vi "Drive Threshold and Half.vi"(0 "X In":dbl, 1 "Drive refnum name":string="RobotDrive", 2 "Send to DB Name":string="Numeric Array", 5 "Y In":dbl, 7 "R In":dbl, 9 "Speed Toggle":bool, 11 "Error In":errorcluster) -> (15 "Error Out":errorcluster)   [LabVIEW 2014]
uses:
  <vilib>/Rock Robotics/WPI/RobotDrive/WPI_RobotDriveGetSetRefNum.vi
  <vilib>/Rock Robotics/WPI/RobotDrive/WPI_RobotDriveMecanumDrive_Cartesian.vi
  <vilib>/Rock Robotics/Network Tables/SD Write Numeric Array.vi
panel:
  out "X Original":dbl
  out "X Threshold":dbl
  out "Y Original":dbl
  out "Y Threshold":dbl
  out "R Original":dbl
  out "R Threshold":dbl
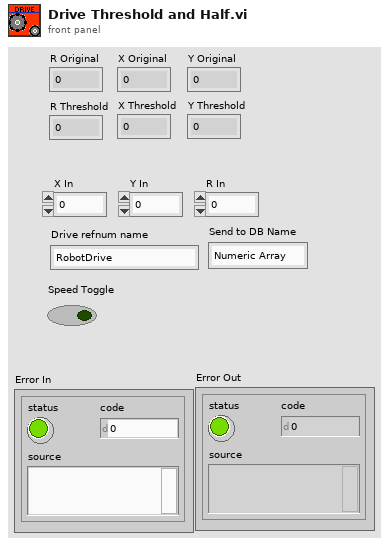
[diagram p1: front panel]
types:
  T1 = typedef "WPI_RobotDriveDevRef.ctl" = cluster{"DevStatus":errorcluster, "Motors[]":T2[], "Square Inputs":bool, "Max Output":dbl}
  T2 = typedef "WPI_MotorControlDeviceRef.ctl" = cluster{"DeviceStatus":errorcluster, "Type":T3, "PWM":cluster{"Controller":T4, "PWM Channel":T5, "DeadBand":T6}, "CAN":cluster{"Device Number":u8, "Control Mode":T7, "Semaphore":T8, "Max Vout":dbl, "TalonSRX Control Mode":T9}, "Invert":bool, "TransformRef":T10, "InvTransformRef":T10}
  T3 = typedef "WPI_MotorControlType.ctl" = enum16{"PWM", "CAN", "CANTalonSRX"}
  T4 = typedef "FPGA_TypedefDigitalModule.ctl" = enum16{"Controller 1"}
  T5 = typedef "FPGA_DIOPWMChannel.ctl" = enum8{"PWM 0", "PWM 1", "PWM 2", "PWM 3", "PWM 4", "PWM 5", "PWM 6", "PWM 7", "PWM 8", "PWM 9", "PWM MXP 0", "PWM MXP 1", "PWM MXP 2", "PWM MXP 3", "PWM MXP 4", "PWM MXP 5", "PWM MXP 6", "PWM MXP 7", "PWM MXP 8", "PWM MXP 9", "Invalid"}
  T6 = typedef "WPI_PWMDeadband.ctl" = cluster{"Name":string, "maxPositivePwm":i32, "minPositivePwm":i32, "centerPwm":i32, "maxNegativePwm":i32, "minNegativePwm":i32, "angularRange":u16}
  T7 = typedef "WPI_CANJaguar_ControlMode.ctl" = enum8{"Percent VBus", "Current", "Speed", "Position", "Voltage"}
  T8 = typedef "Semaphore RefNum" = refnum<k1>
  T9 = typedef "WPI_CANTalonSRX_APIControlMode.ctl" = enum8{"Percent VBus", "Speed", "Position", "Slave", "Unchanged / Invalid"}
  T10 = typedef "WPI_PWMTransform_ConPane.ctl" = refnum<vi>
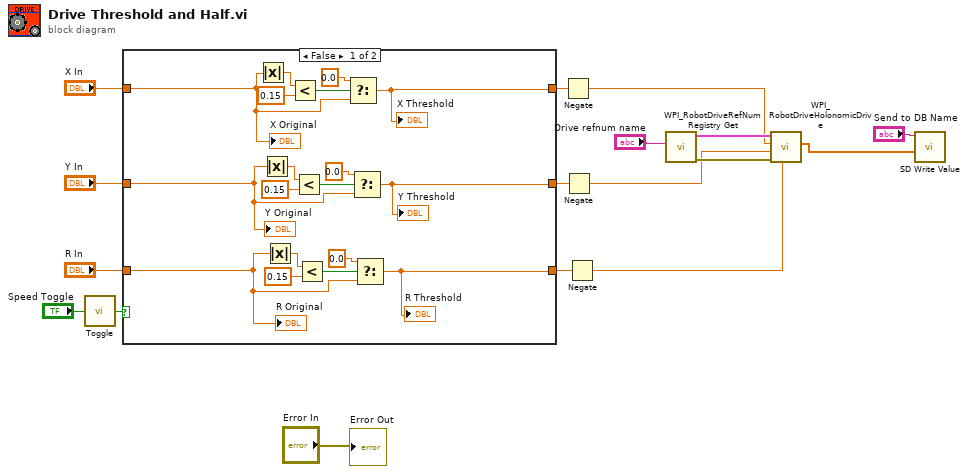
[diagram p0: block diagram]
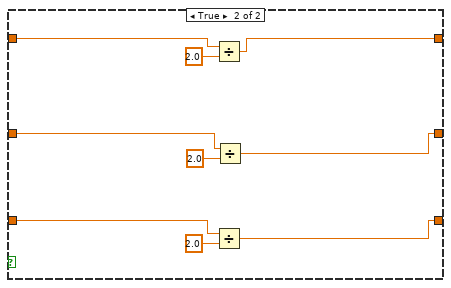
[diagram p2: hidden frame]
diagram:
  n1 = call "Toggle.vi"("Input"="Speed Toggle") -> ("Output"=w17:bool)
  n2 = case shown="False" w17 {
    tunnel: [w30 w38] -> w16
    tunnel: "X In" -> [w31 w39]
    tunnel: "Y In" -> [w25 w40]
    tunnel: [w24 w37] -> w11
    tunnel: "R In" -> [w19 w41]
    tunnel: [w18 w36] -> w10
    frame False {
      n3 = Absolute Value(x=w31) -> (abs(x)=w35:dbl)
      n4 = Absolute Value(x=w25) -> (abs(x)=w29:dbl)
      n5 = Absolute Value(x=w19) -> (abs(x)=w20:dbl)
      n6 = Less?(x=w35, y=0.15) -> (x < y?=w33:bool)
      n7 = Less?(x=w29, y=0.15) -> (x < y?=w27:bool)
      n8 = Less?(x=w20, y=0.15) -> (x < y?=w22:bool)
      n9 = Select(t=0.0, s=w33, f=w31) -> (s? t:f=w30:dbl)
      "X Threshold" <- w30
      n10 = Select(t=0.0, s=w27, f=w25) -> (s? t:f=w24:dbl)
      "Y Threshold" <- w24
      n11 = Select(t=0.0, s=w22, f=w19) -> (s? t:f=w18:dbl)
      "R Threshold" <- w18
      "X Original" <- w31
      "Y Original" <- w25
      "R Original" <- w19
    }
    frame True {
      n12 = Divide(x=w39, y=2.0) -> (x/y=w38:dbl)
      n13 = Divide(x=w41, y=2.0) -> (x/y=w36:dbl)
      n14 = Divide(x=w40, y=2.0) -> (x/y=w37:dbl)
    }
  }
  n15 = Negate(x=w16) -> (-x=w4:dbl)
  n16 = Negate(x=w11) -> (-x=w3:dbl)
  n17 = Negate(x=w10) -> (-x=w2:dbl)
  n18 = call <vilib>:"WPI_RobotDriveRefNum Registry Get.vi"("refnum name"="Drive refnum name") -> ("error out"=w9:errorcluster, "RobotDriveDevRef"=w8:T1)  [unwired: 9 in]
  n19 = call-poly <vilib>:"WPI_RobotDriveHolonomicDrive.vi"("Rotation"=w2, "error in (no error)"=w9, "Y"=w3, "X"=w4, "RobotDriveDevRef"=w8) -> ("Motor Values"=w7:dbl[])  [unwired: 4 in, 2 out]
  n20 = call-poly <vilib>:"SD Write Value.vi"("Numeric Array"=w7, "Name"="Send to DB Name") -> ()  [unwired: 8 in, 2 out]
  "Error Out" <- "Error In"
